vi "Teleop.vi"(10 "Match Info":T1={"Autonomous Elapsed Seconds"=0.0, "TeleOp Elapsed Seconds"=0.0, "Disabled Elapsed Seconds"=0.0, "Visited Autonomous"=FALSE, "Visited TeleOp"=FALSE, "Visited Disabled"=FALSE, "Autonomous Settings"={"Autonomous Style"=enum."Independent", "VI Refnum"=refnum}}, 11 "Call Context":T2) -> ()   [LabVIEW 2017]
doc: "This VI is called for each TeleOp packet received from the DS where the robot is not disabled. It is often used to read from the joysticks and update I/O or to update setpoints for timed control loops. It should complete and return within 20 milliseconds or it may miss DS packets."
uses:
  <vilib>/Rock Robotics/WPI/DriverStation/WPI_DriverStationDerivedRobotMode.ctl
  <vilib>/Rock Robotics/WPI/DriverStation/WPI_DriverStationMatch Info.ctl
  <vilib>/Rock Robotics/WPI/Solenoid/WPI_SolenoidValue.ctl
  <vilib>/Rock Robotics/WPI/ThirdParty/Phoenix-LabVIEW/Motor Controller/Controls/CTRE_Phoenix_MotorControl_ControlMode.ctl
  <vilib>/Rock Robotics/WPI/Utilities/WPI_GetSetVariantRefNum.vi
  <vilib>/Rock Robotics/Network Tables/NT Write Boolean.vi
  <vilib>/Rock Robotics/Network Tables/NT Write Numeric Array.vi
  <vilib>/Rock Robotics/Network Tables/NT Write Boolean Array.vi
  <vilib>/Rock Robotics/WPI/Solenoid/WPI_SolenoidSetEnum.vi
panel:
  out "SHooter speed scale":dbl
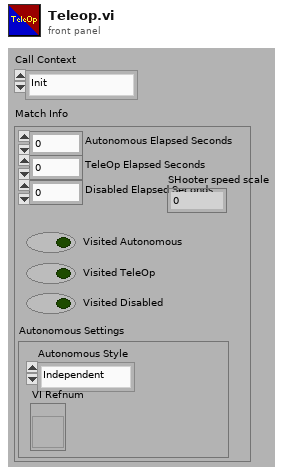
[diagram p1: front panel]
types:
  T1 = typedef "WPI_DriverStationMatch Info.ctl" = cluster{"Autonomous Elapsed Seconds":dbl, "TeleOp Elapsed Seconds":dbl, "Disabled Elapsed Seconds":dbl, "Visited Autonomous":bool, "Visited TeleOp":bool, "Visited Disabled":bool, "Autonomous Settings":cluster{"Autonomous Style":enum16{"Iterative", "Independent"}, "VI Refnum":refnum<vi>}}
  T2 = typedef "WPI_DriverStationDerivedRobotMode.ctl" = enum16{"Init", "Execute", "Stop"}
  T3 = typedef "CTRE_Phoenix_MotorControl_ControlMode.ctl" = u16
  T4 = typedef "WPI_SolenoidValue.ctl" = enum16{"Off", "On", "Forward", "Reverse"}
  T5 = typedef "WPI_CompressorDevRef.ctl" = cluster{"DevStatus":errorcluster, "Pneumatics Control Module":u8}
  T6 = cluster{"Buttons[0]":bool, "Buttons[1]":bool, "Buttons[2]":bool, "Buttons[3]":bool, "Buttons[4]":bool, "Buttons[5]":bool, "Buttons[6]":bool, "Buttons[7]":bool, "Buttons[8]":bool}
  T7 = cluster{"Axes[0]":dbl, "Axes[1]":dbl, "Axes[2]":dbl, "Axes[3]":dbl, "Axes[4]":dbl, "Axes[5]":dbl, "Axes[6]":dbl, "Axes[7]":dbl, "Axes[8]":dbl}
  T8 = typedef "WPI_DriverStationAllianceInfo.ctl" = enum16{"Red", "Blue", "Invalid"}
  T9 = typedef "WPI_RobotDriveDevRef.ctl" = cluster{"DevStatus":errorcluster, "Motors[]":T10[], "Square Inputs":bool, "Max Output":dbl}
  T10 = typedef "WPI_MotorControlDeviceRef.ctl" = cluster{"DeviceStatus":errorcluster, "Type":T11, "PWM":cluster{"PWM Channel":T12, "DeadBand":T13}, "CAN":cluster{"Device Number":u8, "SetOutput VI Ref":variant, "GetOutput VI Ref":variant, "Enable VI Ref":variant, "Disable VI Ref":variant, "Data":variant}, "Invert":bool, "DIO PWM":cluster{"PWM \"Enable\" Channel":T12, "DIOChannel":T14, "PWM Rate":dbl}}
  T11 = typedef "WPI_MotorControlType.ctl" = enum16{"PWM", "CAN", "DIO PWM"}
  T12 = typedef "FPGA_DIOPWMChannel.ctl" = enum8{"PWM 0", "PWM 1", "PWM 2", "PWM 3", "PWM 4", "PWM 5", "PWM 6", "PWM 7", "PWM 8", "PWM 9", "PWM MXP 0", "PWM MXP 1", "PWM MXP 2", "PWM MXP 3", "PWM MXP 4", "PWM MXP 5", "PWM MXP 6", "PWM MXP 7", "PWM MXP 8", "PWM MXP 9", "Invalid"}
  T13 = typedef "WPI_PWMDeadband.ctl" = cluster{"Name":string, "maxPositivePwm":i32, "minPositivePwm":i32, "centerPwm":i32, "maxNegativePwm":i32, "minNegativePwm":i32, "angularRange":u16}
  T14 = typedef "FPGA_DIOChannel.ctl" = enum8{"DIO 0", "DIO 1", "DIO 2", "DIO 3", "DIO 4", "DIO 5", "DIO 6", "DIO 7", "DIO 8", "DIO 9", "DIO MXP 0", "DIO MXP 1", "DIO MXP 2", "DIO MXP 3", "DIO MXP 4", "DIO MXP 5", "DIO MXP 6", "DIO MXP 7", "DIO MXP 8", "DIO MXP 9", "DIO MXP 10", "DIO MXP 11", "DIO MXP 12", "DIO MXP 13", "DIO MXP 14", "DIO MXP 15", "SPI Port CS1", "SPI Port CS2", "SPI Port CS3", "SPI Port MISO", "SPI Port MOSI", "Invalid"}
  T15 = typedef "WPI_SolenoidDevRef.ctl" = cluster{"DevStatus":errorcluster, "Pneumatics Control Module":u8, "Forward Solenoid Channel":T16, "Reverse Solenoid Channel":T16}
  T16 = typedef "WPI_SolenoidChannel.ctl" = enum8{"Solenoid 0", "Solenoid 1", "Solenoid 2", "Solenoid 3", "Solenoid 4", "Solenoid 5", "Solenoid 6", "Solenoid 7", "Invalid"}
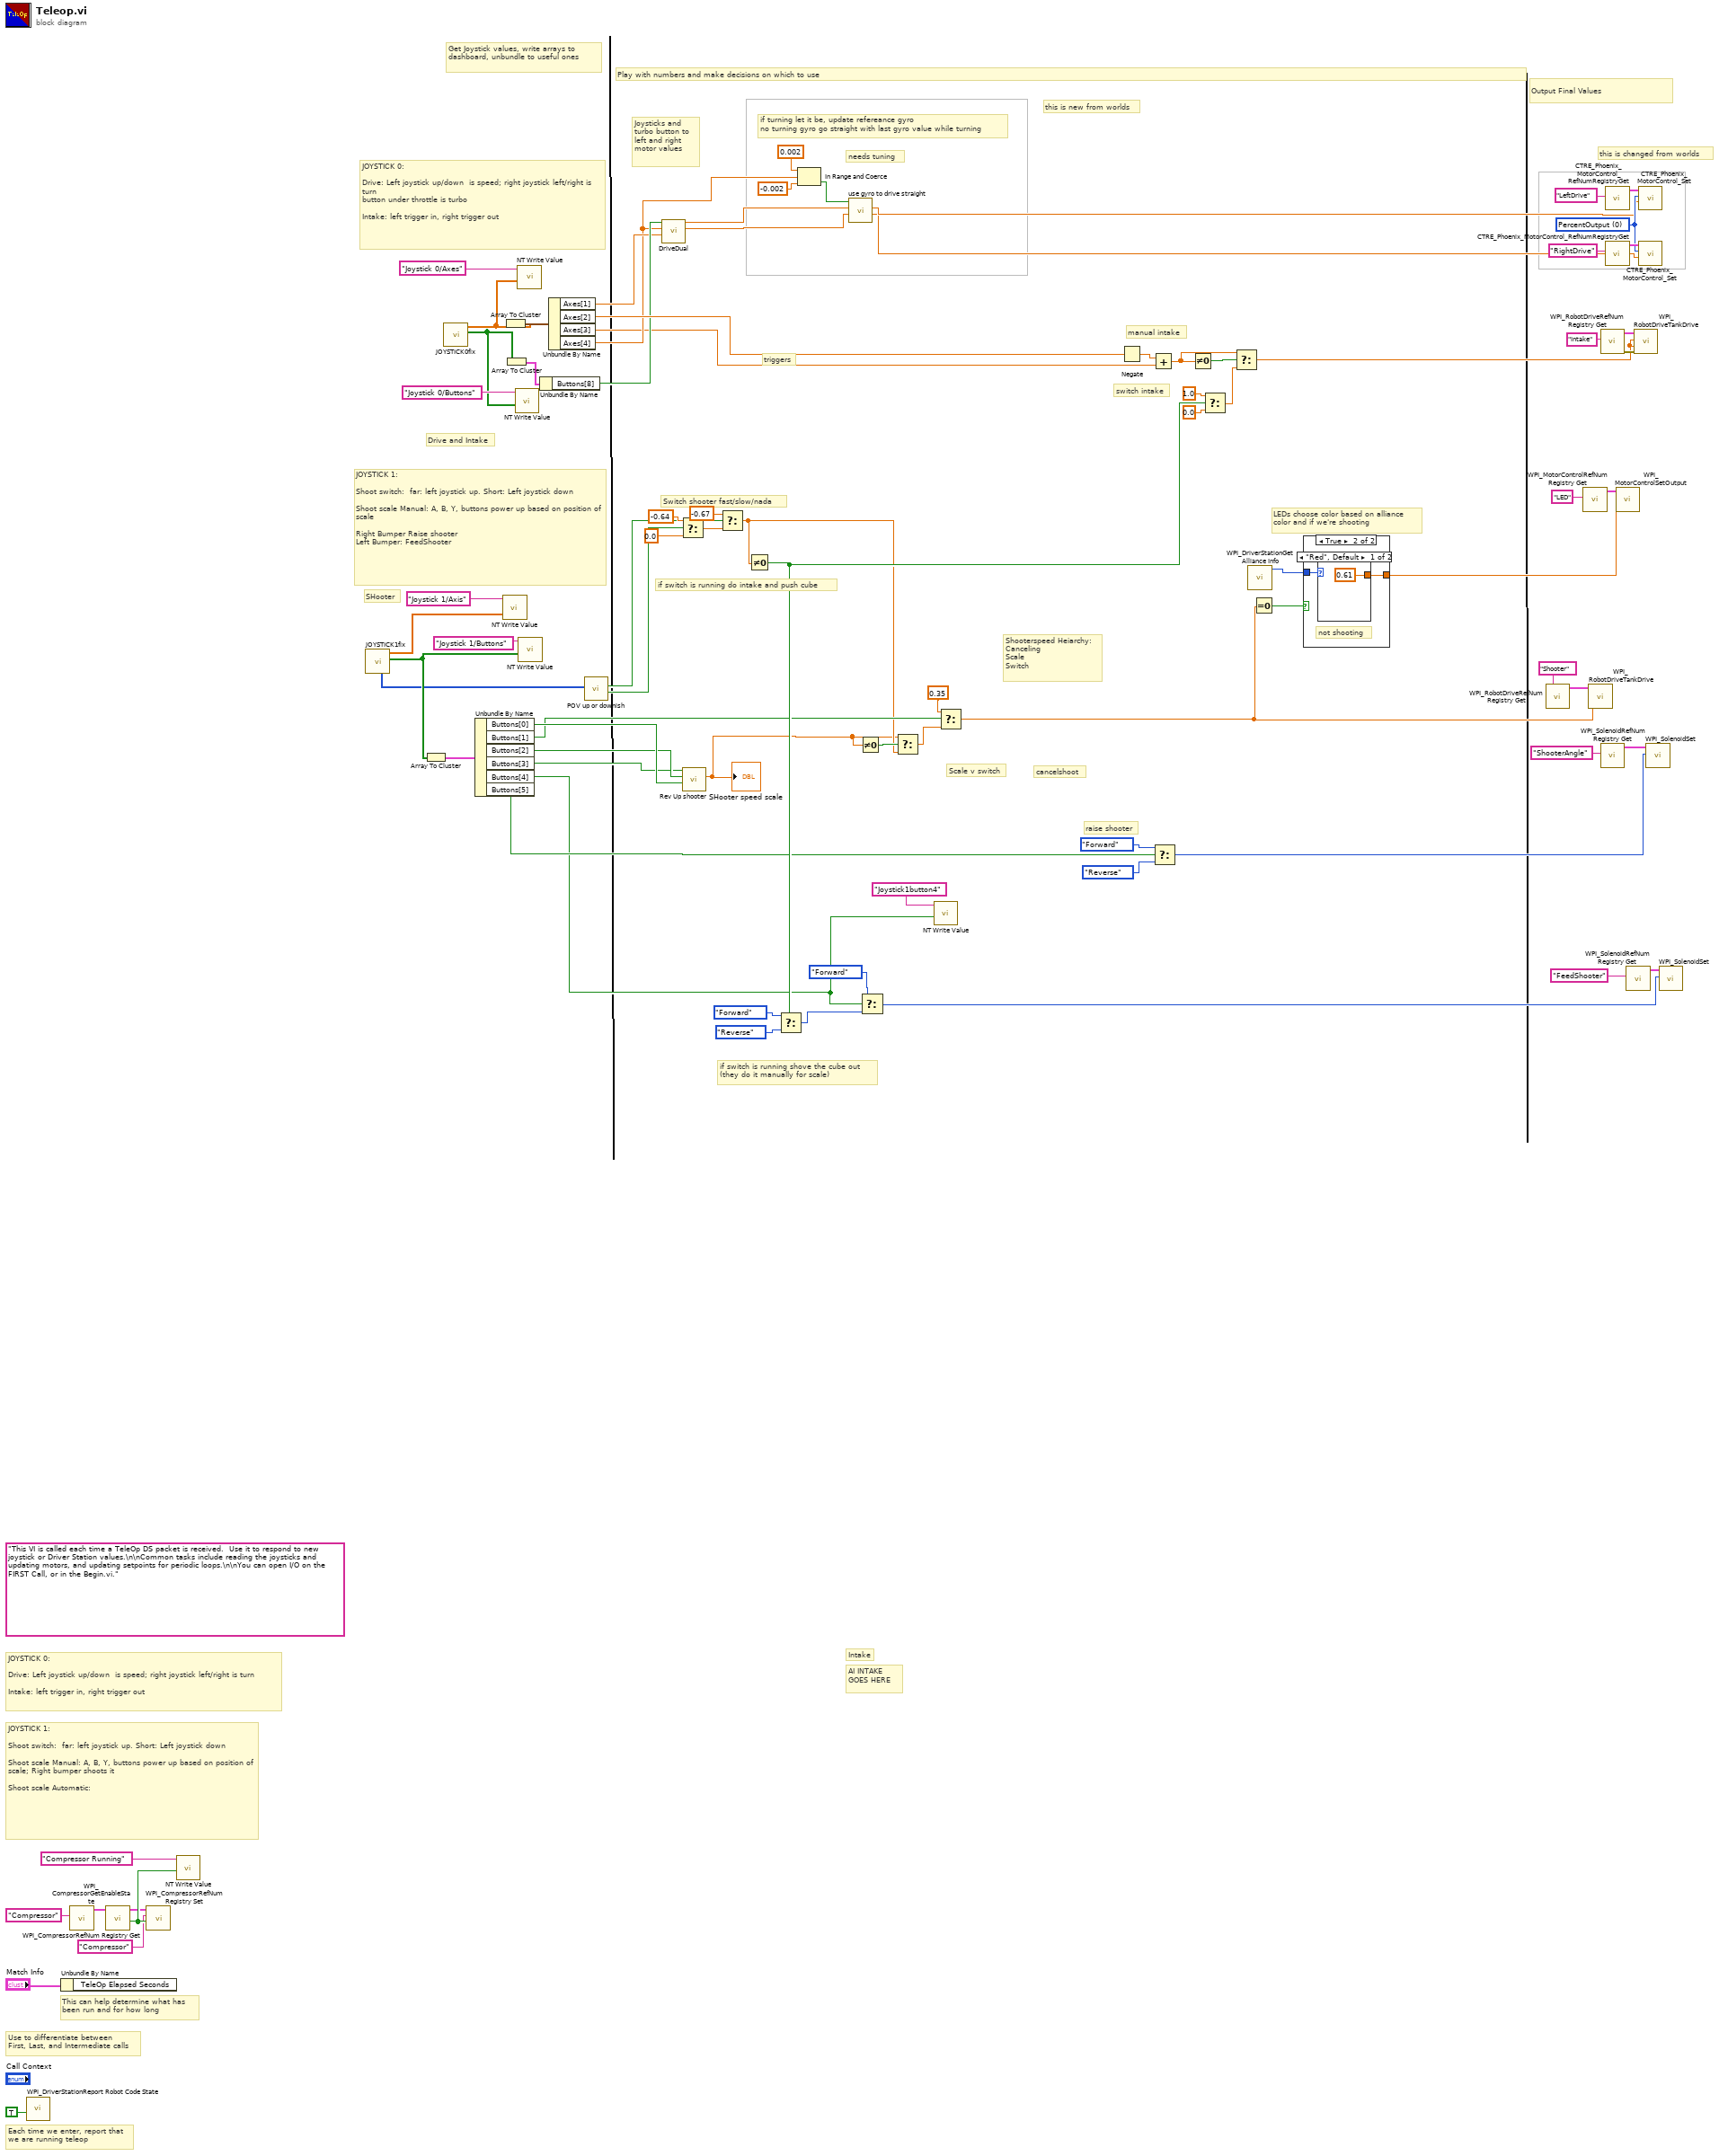
[diagram p0: block diagram]
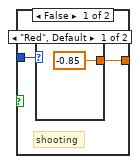
[diagram p2: hidden frame]
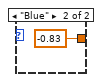
[diagram p3: hidden frame]
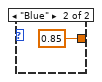
[diagram p4: hidden frame]
diagram:
  w13 = T3 0 items=["PercentOutput"=0, "Position"=1, "Velocity"=2, "Current"=3, "Follower"=5, "MotionProfile"=6, "MotionMagic"=7, "MotionMagicArc"=8, "MotionProfileArc"=10, "Disabled"=15] ("Control Mode")
  (unwired) "This VI is called each time a TeleOp DS packet is received.  Use it to respond to new joystick or Driver Station values.\n\nCommon tasks include reading the joysticks and updating motors, and updating setpoints for periodic loops.\n\nYou can open I/O on the FIRST Call, or in the Begin.vi."
  # "if switch is running do intake and push cube"
  # "if switch is running shove the cube out\n(they do it manually for scale)"
  # "Scale v switch"
  # "Shooterspeed Heiarchy:\nCanceling\nScale\nSwitch"
  # "raise shooter"
  # "LEDs choose color based on alliance color and if we're shooting"
  # "triggers"
  # "this is changed from worlds"
  # "this is new from worlds"
  # "needs tuning"
  # "Play with numbers and make decisions on which to use"
  # "Joysticks and turbo button to left and right motor values"
  # "Output Final Values"
  # "Get Joystick values, write arrays to dashboard, unbundle to useful ones"
  # "if turning let it be, update refereance gyro\nno turning gyro go straight with last gyro value while turning"
  # "SHooter"
  # "cancelshoot"
  # "Switch shooter fast/slow/nada"
  # "switch intake"
  # "manual intake"
  # "Drive and Intake"
  # "JOYSTICK 1:\n\nShoot switch:  far: left joystick up. Short: Left joystick down\n\nShoot scale Manual: A, B, Y, buttons power up based on position of scale\n\nRight Bumper Raise shooter\nLeft Bumper: FeedShooter"
  # "JOYSTICK 0:\n\nDrive: Left joystick up/down  is speed; right joystick left/right is turn\nbutton under throttle is turbo\n\nIntake: left trigger in, right trigger out"
  # "AI INTAKE GOES HERE"
  # "Intake"
  # "JOYSTICK 1:\n\nShoot switch:  far: left joystick up. Short: Left joystick down\n\nShoot scale Manual: A, B, Y, buttons power up based on position of scale; Right bumper shoots it \n\nShoot scale Automatic:"
  # "JOYSTICK 0:\n\nDrive: Left joystick up/down  is speed; right joystick left/right is turn\n\nIntake: left trigger in, right trigger out"
  # "Each time we enter, report that\nwe are running teleop"
  # "Use to differentiate between\nFirst, Last, and Intermediate calls"
  # "This can help determine what has\nbeen run and for how long"
  n1 = call <vilib>:"WPI_DriverStationReport Robot Code State.vi"("TeleOp"=TRUE ("Autonomous")) -> ()  [unwired: 10 in, 1 out]
  n2 = Unbundle By Name("Match Info") -> ()  [unwired: 1 out]
  n3 = call <vilib>:"WPI_CompressorRefNum Registry Get.vi"("refnum name"="Compressor") -> ("CompressorDevRef"=w80:T5)  [unwired: 9 in, 1 out]
  n4 = call <vilib>:"WPI_CompressorGetEnableState.vi"("CompressorDevRef"=w80) -> ("Compressor Running"=w82:bool, "CompressorDevRef"=w81:T5)  [unwired: 7 in, 2 out]
  n5 = call <vilib>:"WPI_CompressorRefNum Registry Set.vi"("Test Mode Only"=w82, "refnum name"="Compressor", "CompressorDevRef"=w81) -> ()  [unwired: 7 in, 2 out]
  n6 = call-poly <vilib>:"NT Write Value.vi"("Boolean"=w82, "Name"="Compressor Running") -> ()  [unwired: 9 in, 1 out]
  n7 = call "JOYSTICK1fix.vi"() -> ("Buttons"=w24:bool[], "Axes"=w23:dbl[], "POVs"=w22:i16[])  [unwired: 8 in, 1 out]
  n8 = Array To Cluster(array=w24) -> (cluster=w65:T6)
  n9 = call "JOYSTICK0fix.vi"() -> ("Buttons"=w27:bool[], "Axes"=w26:dbl[])  [unwired: 8 in, 2 out]
  n10 = Unbundle By Name(w65) -> ("Buttons[0]"=w64:bool, "Buttons[1]"=w20:bool, "Buttons[2]"=w63:bool, "Buttons[3]"=w62:bool, "Buttons[4]"=w18:bool, "Buttons[5]"=w28:bool)
  n11 = call-poly <vilib>:"NT Write Value.vi"("Numeric Array"=w23, "Name"="Joystick 1/Axis") -> ()  [unwired: 9 in, 1 out]
  n12 = Array To Cluster(array=w26) -> (cluster=w61:T7)
  n13 = Array To Cluster(array=w27) -> (cluster=w59:T6)
  n14 = call-poly <vilib>:"NT Write Value.vi"("Boolean Array"=w27, "Name"="Joystick 0/Buttons") -> ()  [unwired: 9 in, 1 out]
  n15 = call-poly <vilib>:"NT Write Value.vi"("Numeric Array"=w26, "Name"="Joystick 0/Axes") -> ()  [unwired: 9 in, 1 out]
  n16 = call-poly <vilib>:"NT Write Value.vi"("Boolean Array"=w24, "Name"="Joystick 1/Buttons") -> ()  [unwired: 9 in, 1 out]
  n17 = Unbundle By Name(w59) -> ("Buttons[8]"=w32:bool)
  n18 = Unbundle By Name(w61) -> ("Axes[1]"=w31:dbl, "Axes[2]"=w60:dbl, "Axes[3]"=w8:dbl, "Axes[4]"=w12:dbl)
  n19 = call "POV up or downish.vi"("POV"=w22) -> ("DOWNish"=w66:bool, "UPish"=w67:bool)  [unwired: 9 in]
  n20 = call "DriveDual.vi"("YAxis"=w31, "XAxis"=w12, "Turbo?"=w32) -> ("Right"=w4:dbl, "Left"=w5:dbl)  [unwired: 7 in]
  n21 = Select(t=-0.64 ("f"), s=w66, f=0.0) -> (s? t:f=w73:dbl)
  n22 = call "Rev Up shooter.vi"("LowSpeed"=w64, "MidSpeed"=w63, "TopSpeed"=w62) -> ("Speed"=w6:dbl)  [unwired: 7 in, 1 out]
  "SHooter speed scale" <- w6
  n23 = Select(t=-0.67, s=w67, f=w73) -> (s? t:f=w7:dbl)
  n24 = Not Equal To 0?(x=w7) -> (x != 0?=w29:bool)
  n25 = Select(t=WPI_SolenoidValue."Forward" ("Value"), s=w29, f=WPI_SolenoidValue."Reverse") -> (s? t:f=w39:T4)
  n26 = In Range and Coerce(upper limit=0.002, x=w12, lower limit=-0.002) -> (In Range?=w1:bool)  [unwired: 1 out]
  n27 = call "use gyro to drive straight.vi"("RightDriveIn"=w4, "LeftDriveIn"=w5, "Trying to go Straight"=w1) -> ("RightDriveOut"=w2:dbl, "LeftDriveOut"=w3:dbl)  [unwired: 7 in]
  n28 = Not Equal To 0?(x=w6) -> (x != 0?=w44:bool)
  n29 = Select(t=WPI_SolenoidValue."Forward" ("Value"), s=w18, f=w39) -> (s? t:f=w38:T4)
  n30 = Select(t=w6, s=w44, f=w7) -> (s? t:f=w43:dbl)
  n31 = call-poly <vilib>:"NT Write Value.vi"("Boolean"=w18, "Name"="Joystick1button4") -> ()  [unwired: 9 in, 1 out]
  n32 = Select(t=0.35, s=w20, f=w43) -> (s? t:f=w9:dbl)
  n33 = Negate(x=w60) -> (-x=w74:dbl)
  n34 = Add(x=w74, y=w8) -> (x+y=w30:dbl)
  n35 = Select(t=WPI_SolenoidValue."Forward" ("Value"), s=w28, f=WPI_SolenoidValue."Reverse" ("Value")) -> (s? t:f=w37:T4)
  n36 = Not Equal To 0?(x=w30) -> (x != 0?=w46:bool)
  n37 = Select(t=1.0, s=w29, f=0.0) -> (s? t:f=w25:dbl)
  n38 = Select(t=w30, s=w46, f=w25) -> (s? t:f=w45:dbl)
  n39 = call <vilib>:"WPI_DriverStationGet Alliance Info.vi"() -> ("Alliance"=w47:T8)  [unwired: 6 in, 5 out]
  n40 = Equal To 0?(x=w9) -> (x = 0?=w34:bool)
  n41 = case shown="True" w34 {
    tunnel: w47 -> [w87 w92]
    tunnel: [w88 w91] -> w35
    frame False {
      # "shooting"
      n42 = case shown="\"Red\", Default" w87 {
        tunnel: [-0.85 -0.83] -> w88
        frame "Red", Default {
        }
        frame "Blue" {
        }
      }
    }
    frame True {
      # "not shooting"
      n43 = case shown="\"Red\", Default" w92 {
        tunnel: [0.61 0.85] -> w91
        frame "Red", Default {
        }
        frame "Blue" {
        }
      }
    }
  }
  n44 = call <vilib>:"WPI_RobotDriveRefNum Registry Get.vi"("refnum name"="Shooter") -> ("RobotDriveDevRef"=w54:T9)  [unwired: 9 in, 1 out]
  n45 = call <vilib>:"WPI_MotorControlRefNum Registry Get.vi"("refnum name"="LED") -> ("MotorControlDevRef"=w48:T10)  [unwired: 9 in, 1 out]
  n46 = call <vilib>:"WPI_RobotDriveTankDrive.vi"("Right axis value"=w9, "Left axis value"=w9, "RobotDriveDevRef"=w54) -> ()  [unwired: 6 in, 3 out]
  n47 = call <vilib>:"WPI_RobotDriveRefNum Registry Get.vi"("refnum name"="Intake") -> ("error out"=w57:errorcluster, "RobotDriveDevRef"=w56:T9)  [unwired: 9 in]
  n48 = call <vilib>:"WPI_SolenoidRefNum Registry Get.vi"("refnum name"="ShooterAngle") -> ("SolenoidDevRef"=w50:T15)  [unwired: 9 in, 1 out]
  n49 = call <vilib>:"CTRE_Phoenix_MotorControl_RefNumRegistryGet.vi"("refnum name"="LeftDrive") -> ("PhoenixMotorControlDevRef"=w17:T10)  [unwired: 9 in, 1 out]
  n50 = call <vilib>:"CTRE_Phoenix_MotorControl_RefNumRegistryGet.vi"("refnum name"="RightDrive") -> ("PhoenixMotorControlDevRef"=w14:T10)  [unwired: 9 in, 1 out]
  n51 = call <vilib>:"WPI_MotorControlSetOutput.vi"("Output"=w35, "MotorControlDevRef"=w48) -> ()  [unwired: 7 in, 3 out]
  n52 = call <vilib>:"WPI_SolenoidRefNum Registry Get.vi"("refnum name"="FeedShooter") -> ("SolenoidDevRef"=w51:T15)  [unwired: 9 in, 1 out]
  n53 = call <vilib>:"WPI_RobotDriveTankDrive.vi"("error in (no error)"=w57, "Right axis value"=w45, "Left axis value"=w45, "RobotDriveDevRef"=w56) -> ()  [unwired: 5 in, 3 out]
  n54 = call <vilib>:"CTRE_Phoenix_MotorControl_Set.vi"("Output"=w3, "Control Mode"=w13, "PhoenixMotorControlDevRef"=w17) -> ()  [unwired: 7 in, 2 out]
  n55 = call <vilib>:"CTRE_Phoenix_MotorControl_Set.vi"("Output"=w2, "Control Mode"=w13, "PhoenixMotorControlDevRef"=w14) -> ()  [unwired: 7 in, 2 out]
  n56 = call-poly <vilib>:"WPI_SolenoidSet.vi"("Value"=w37, "SolenoidDevRef"=w50) -> ()  [unwired: 8 in, 2 out]
  n57 = call-poly <vilib>:"WPI_SolenoidSet.vi"("Value"=w38, "SolenoidDevRef"=w51) -> ()  [unwired: 8 in, 2 out]
